vi "Main.vi"() -> ()   [LabVIEW 2017]
uses:
  1. CTL/DAQ_AO.ctl
  1. CTL/Controller.ctl
  <vilib>/Analysis/3filter.llb/Filter Passband Type.ctl
  <vilib>/DAQmx/read.llb/DAQmx Read (Analog 1D DBL 1Chan NSamp).vi
  <vilib>/DAQmx/write.llb/DAQmx Write (Digital Bool 1Line 1Point).vi
  <vilib>/DAQmx/write.llb/DAQmx Write (Analog 2D DBL NChan NSamp).vi
  <vilib>/DAQmx/create/channels.llb/DAQmx Create Channel (AO-Voltage-Basic).vi
  <vilib>/DAQmx/create/channels.llb/DAQmx Create Channel (AI-Voltage-Basic).vi
  <vilib>/DAQmx/configure/timing.llb/DAQmx Timing (Sample Clock).vi
  <vilib>/DAQmx/create/channels.llb/DAQmx Create Channel (DO-Digital Output).vi
  <vilib>/DAQmx/miscellaneous.llb/DAQmx Fill In Error Info.vi
  <vilib>/Analysis/2dsp.llb/1D Cross Correlation (DBL).vi
  <vilib>/measure/maspectr.llb/FFT Power Spectrum and PSD for 1 Chan.vi
  <vilib>/Analysis/3filter.llb/FIR Windowed Filter (DBL).vi
  <vilib>/Analysis/NI_AALPro.lvlib
  <vilib>/measure/NI_MAPro.lvlib
  <vilib>/Analysis/NI_AALBase.lvlib
panel:
  out "신호처리[1,-1][최대값":dbl
  out "신호처리[1.-1][필터후]":waveform(dbl)(graph)
  out "신호처리[1,-1,][필터후 주파수]":cluster{"f0":dbl, "df":dbl, "magnitude":dbl[]}(graph)
  out "신호처리[1,-1,][주파수]":cluster{"f0":dbl, "df":dbl, "magnitude":dbl[]}(graph)
  out "신호처리[1.-1]":waveform(dbl)(graph)
  in  "Tab Control":T1(tab)
  in  "Version Check":bool=TRUE
  in  "일시 정지 버튼":bool
  out "수신 신호 파형":waveform(dbl)(graph)
  out "송신 신호생성 파형":waveform(dbl)[](graph)
  out "신호처리파형":waveform(dbl)(graph)
  out "최대값":dbl
  out "이전 최대값":dbl
  out "최대값 차이":dbl
  in  "정지 버튼":bool
  in  "수동시작 버튼":bool
  in  "자동시작 버튼":bool
  in  "Chip_rate_Threshold":u32(knob)=10 scale=0.0..20.0
  in  "Threshold":u32(knob)=10 scale=0.0..20.0
  in  "수신시간":dbl=0.5
  in  "Rc":dbl=5500.0 min=4000.0 step=100.0
  in  "Mask 데이터 참조 경로":string="C:\\Users\\FishingNetID\\Desktop\\TRX_CONTROLLER_SIMULATRO_1.4\\3. TDMS\\Coef8.tdms"
  in  "TX_Period":dbl=3.0
  in  "Mask 길이":enum16{"8 Order", "12 Order"}(ring)
  in  "주소":string="192.168.0.147"
  in  "원격 포트 또는 서비스 이름":u16=10000
  out "원소":T2
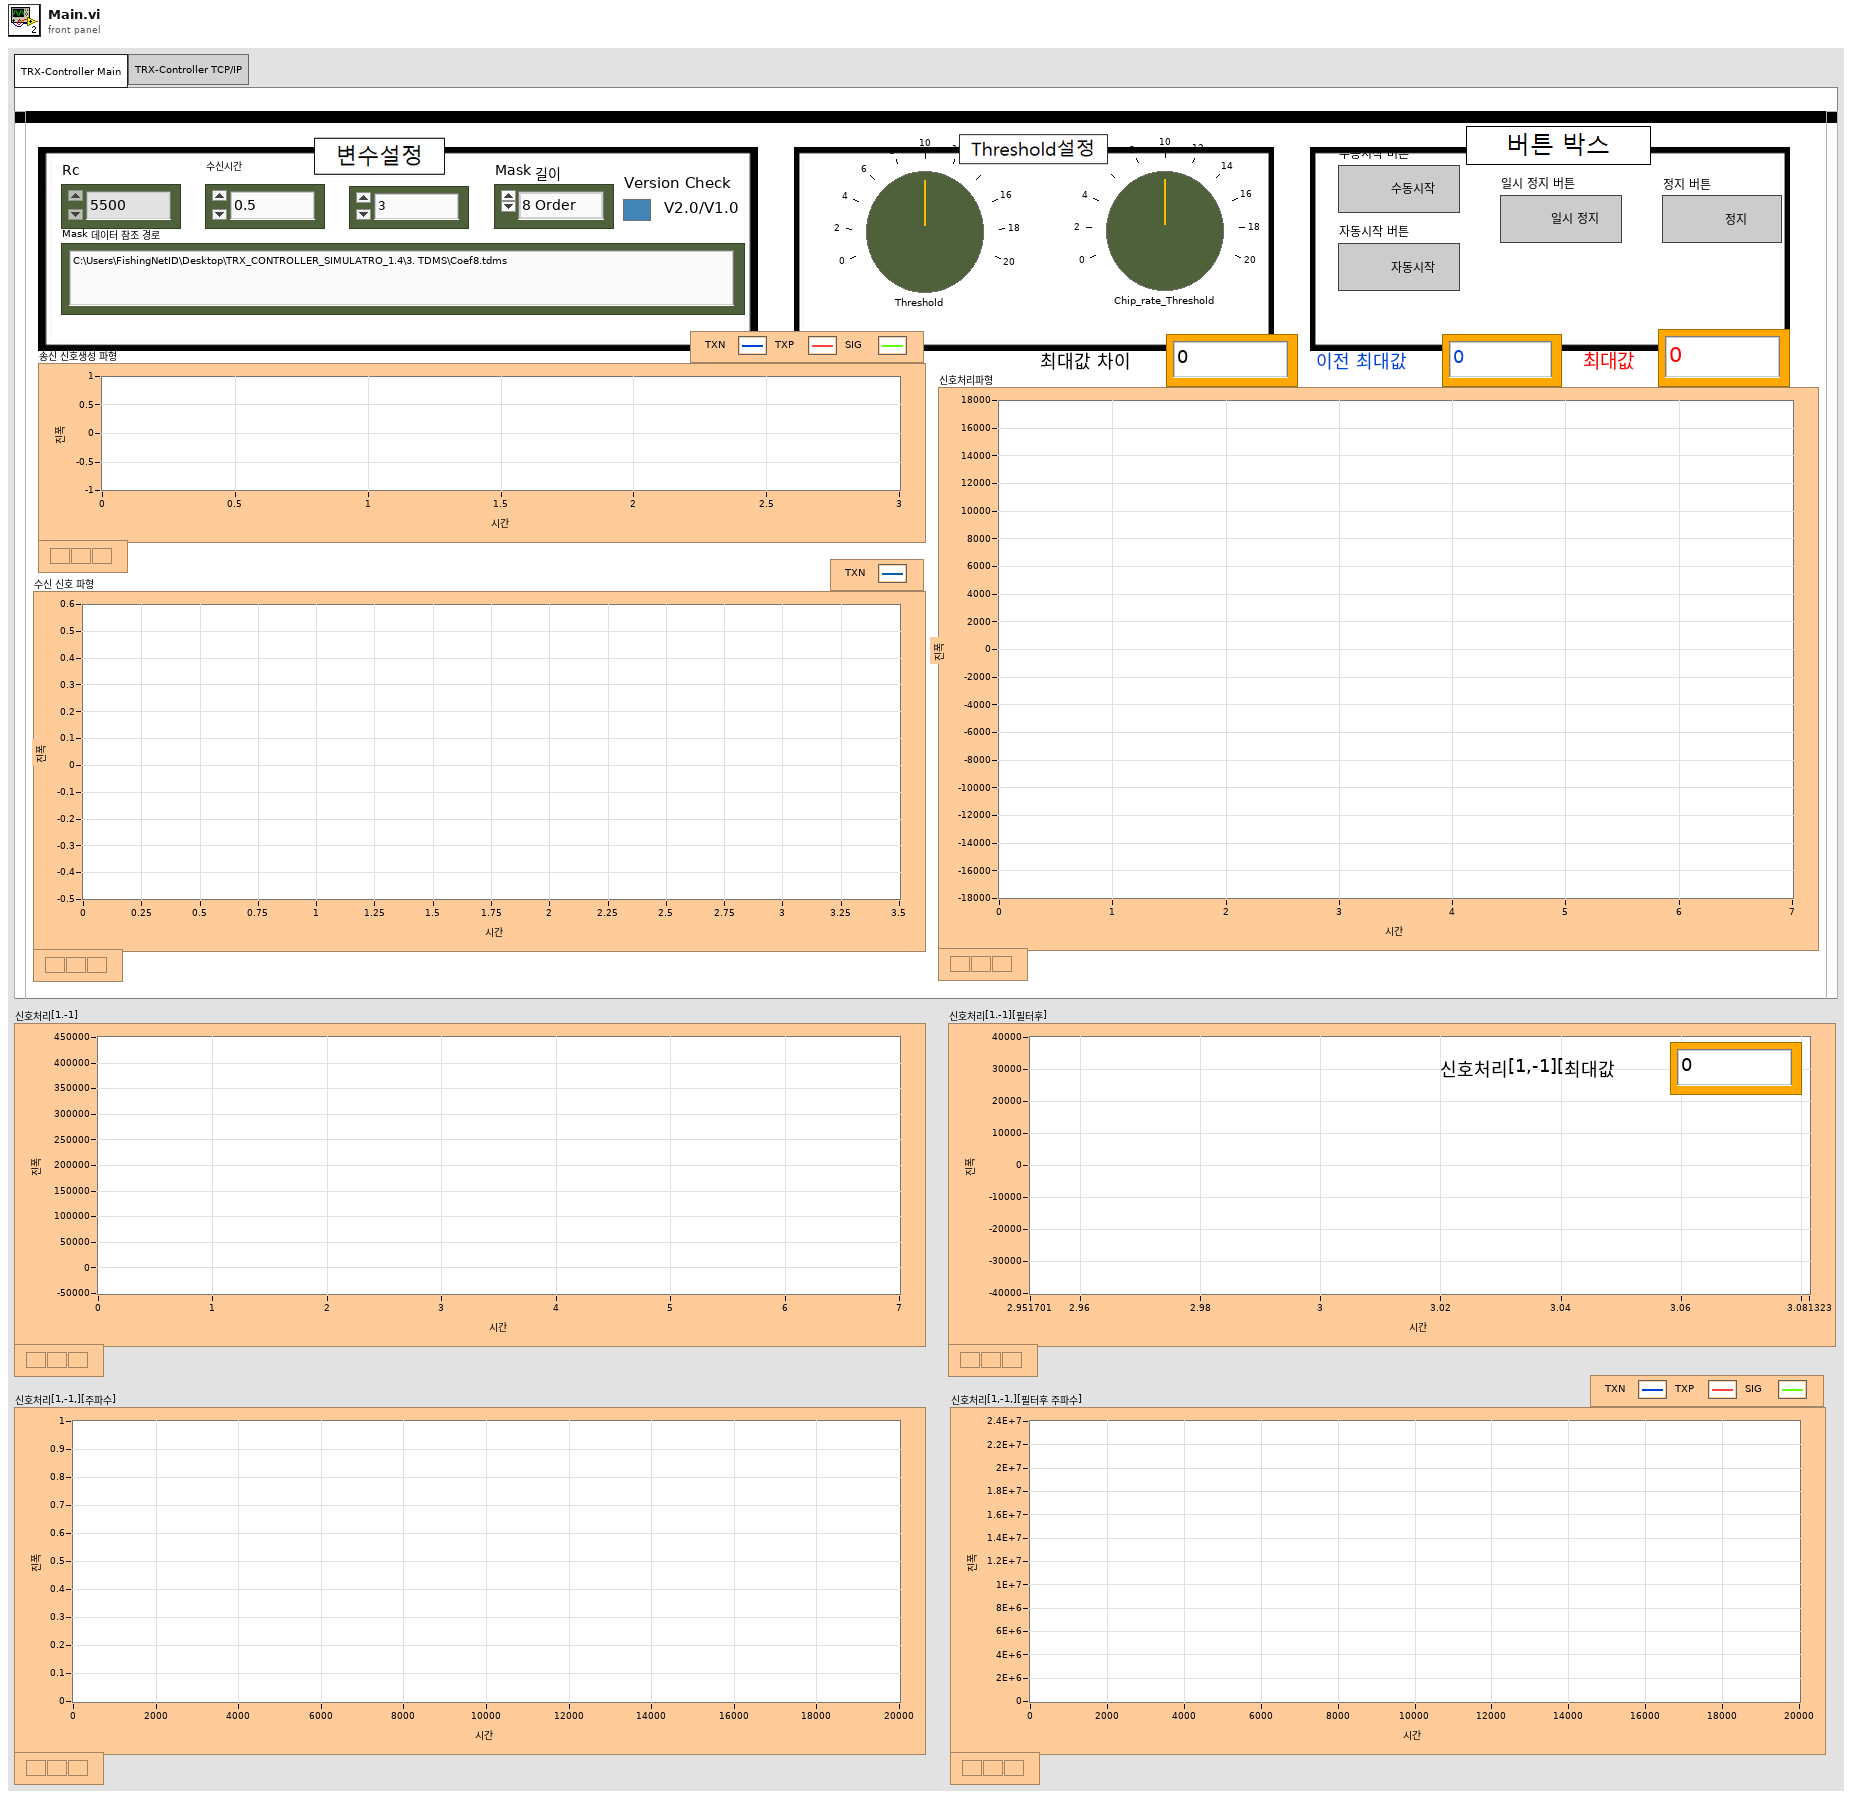
[diagram p1: front panel]
types:
  T1 = enum32{"TRX-Controller Main", "TRX-Controller TCP/IP"}
  T2 = typedef "DAQ_AO.ctl" = enum16{"통신 초기화", "통신 시작", "통신 정지"}
  T3 = cluster{"연결 ID":refnum<k5>, "TCP 에러":errorcluster}
  T4 = cluster{"송신신호 생성":waveform(dbl)[], "TXP 신호":dbl[], "TXN 신호":dbl[], "Fs":dbl, "AI 참조":refnum<k21>, "AO 참조":refnum<k21>, "수신시간":dbl, "Rc":dbl, "이전 최대값":dbl, "수신 신호처리 파형":waveform(dbl), "수신 파형":waveform(dbl), "최대값":dbl, "최대값 차이":dbl, "DO 참조":refnum<k21>, "TXEN 신호":bool[], " 신호처리[1,-1]":waveform(dbl), " 신호처리[1,-1][최대값":dbl, " 신호처리[1,-1][주파수]":cluster{"f0":dbl, "df":dbl, "magnitude":dbl[]}, " 신호처리[1,-1][필터 후 주파수]":cluster{"f0":dbl, "df":dbl, "magnitude":dbl[]}, " 신호처리[1,-1][필터후]":waveform(dbl)}
  T5 = typedef "Controller.ctl" = enum16{"초기화", "수동시작", "신호처리", "정지", "값 변경", "일시정지", "자동시작"}
  T6 = typedef "NI_AALBase.lvlib/Filter Passband Type.ctl" = enum32{"Lowpass", "Highpass", "Bandpass", "Bandstop"}
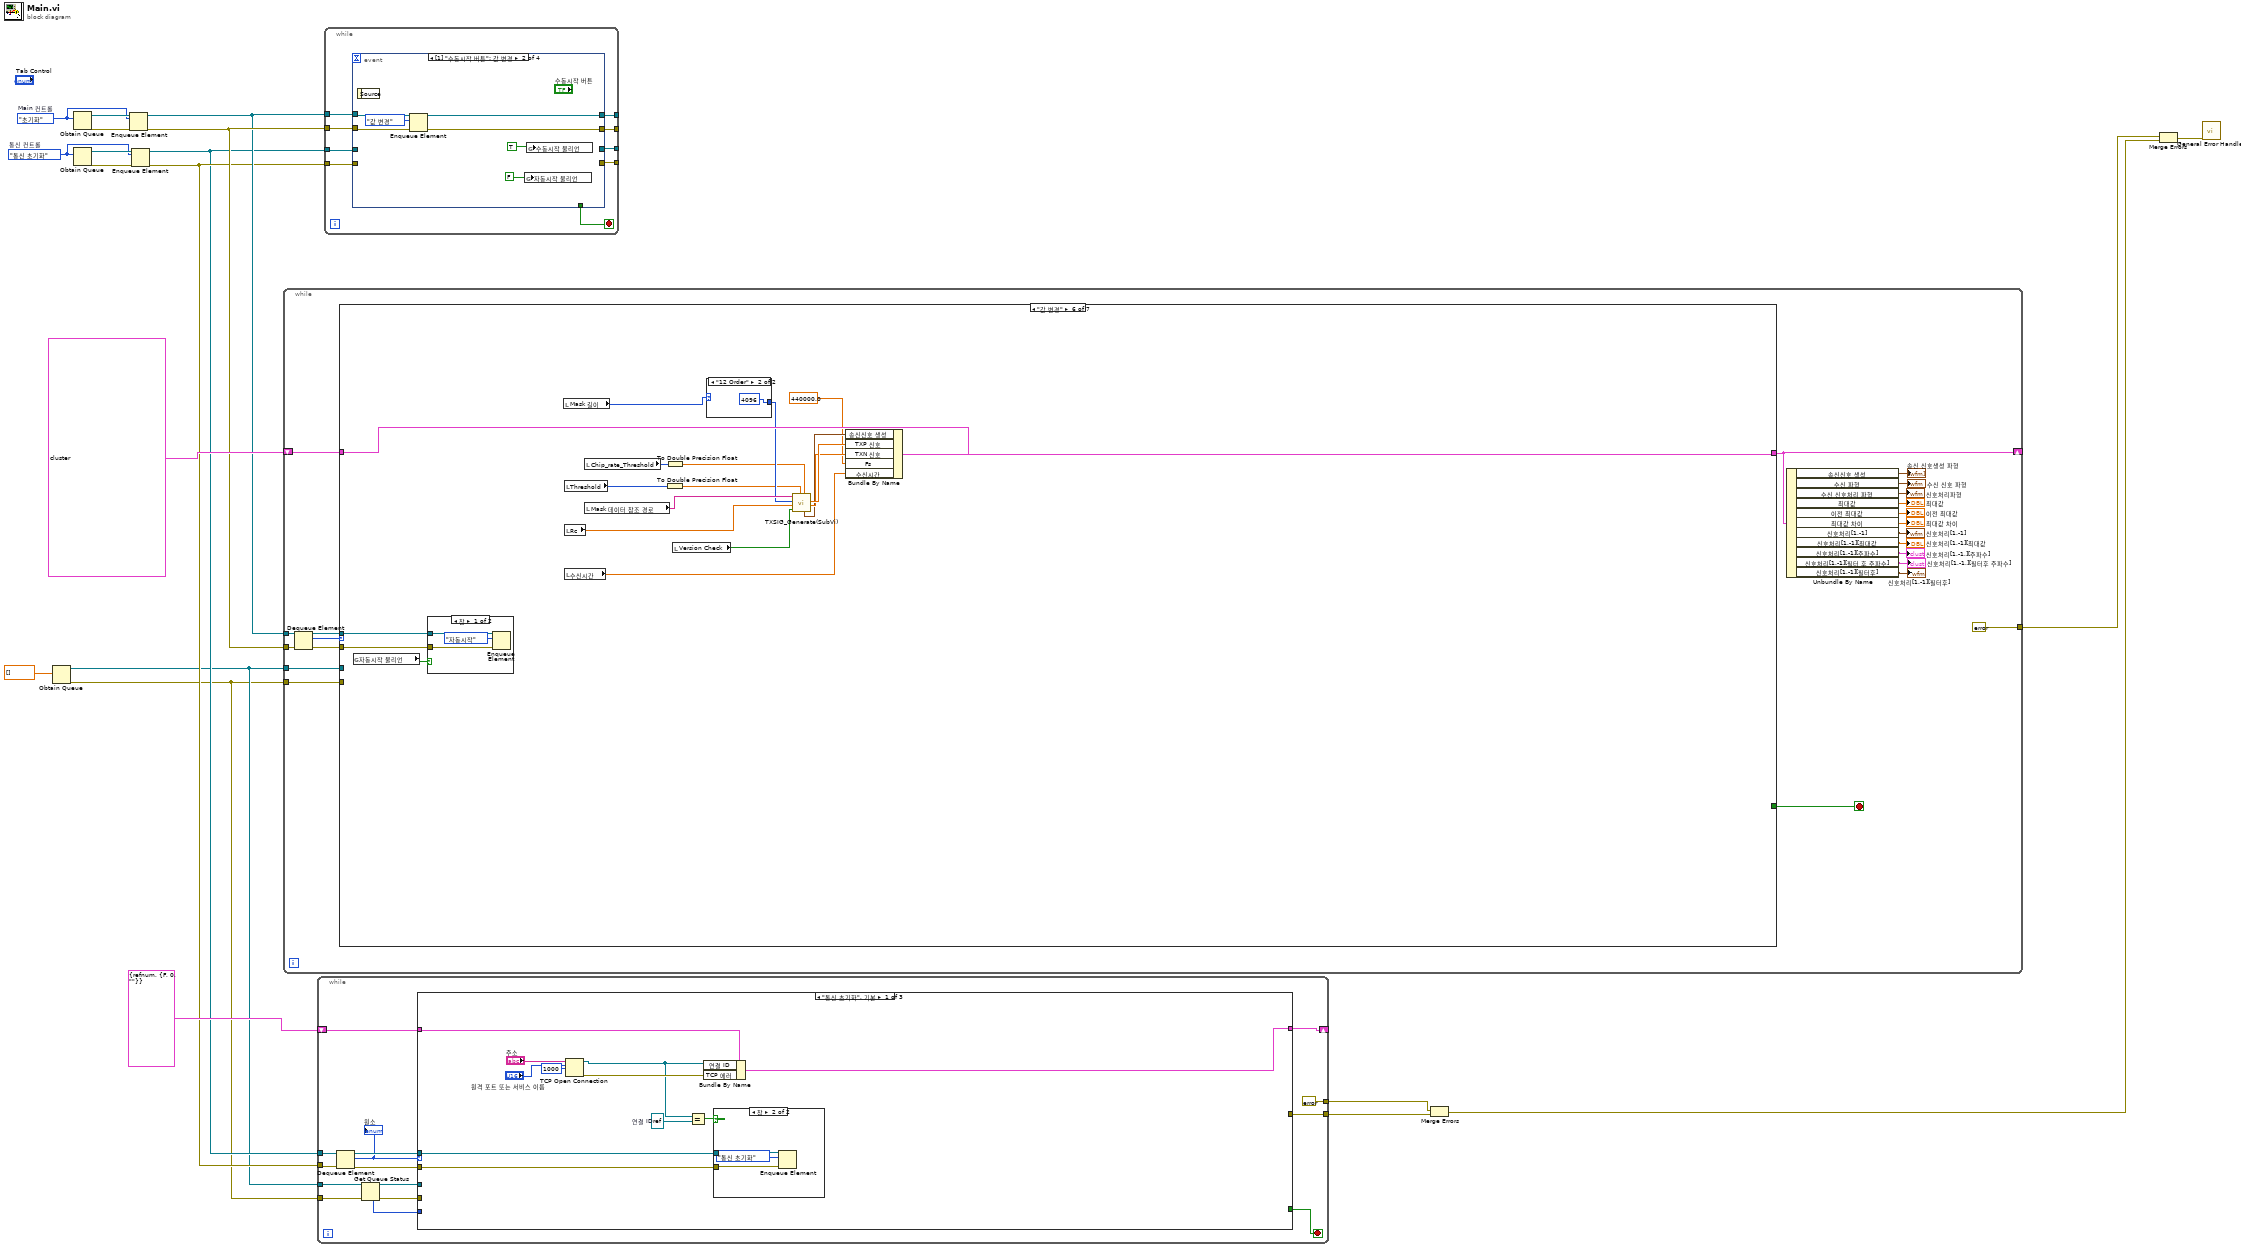
[diagram p0: block diagram]
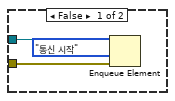
[diagram p2: hidden frame]
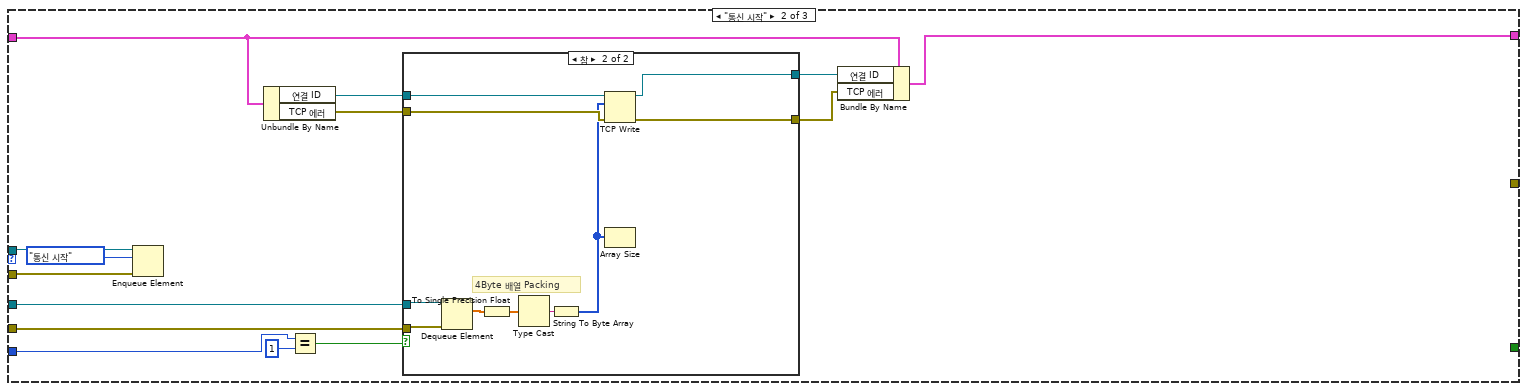
[diagram p3: hidden frame]
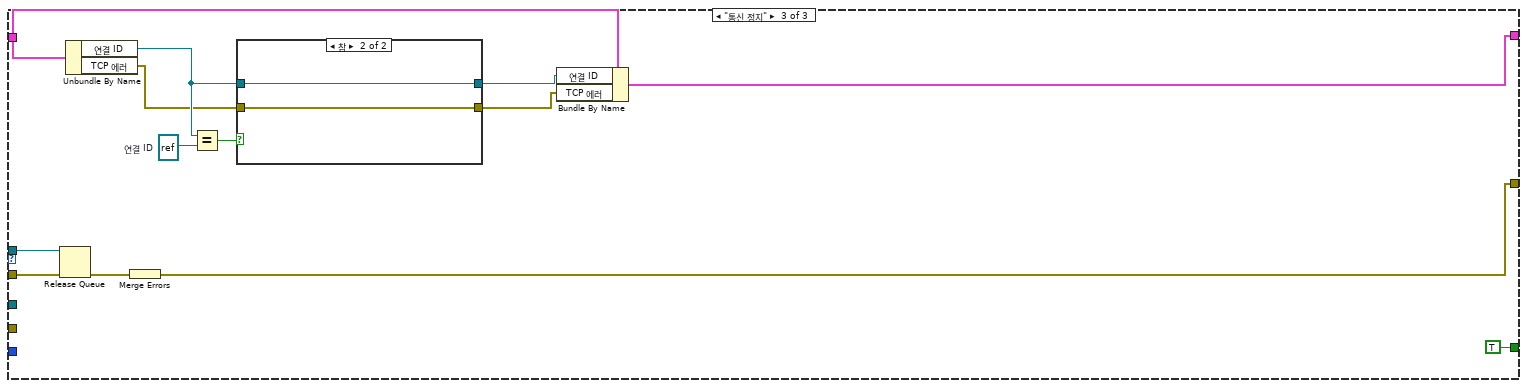
[diagram p5: hidden frame]
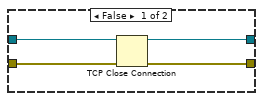
[diagram p6: hidden frame]
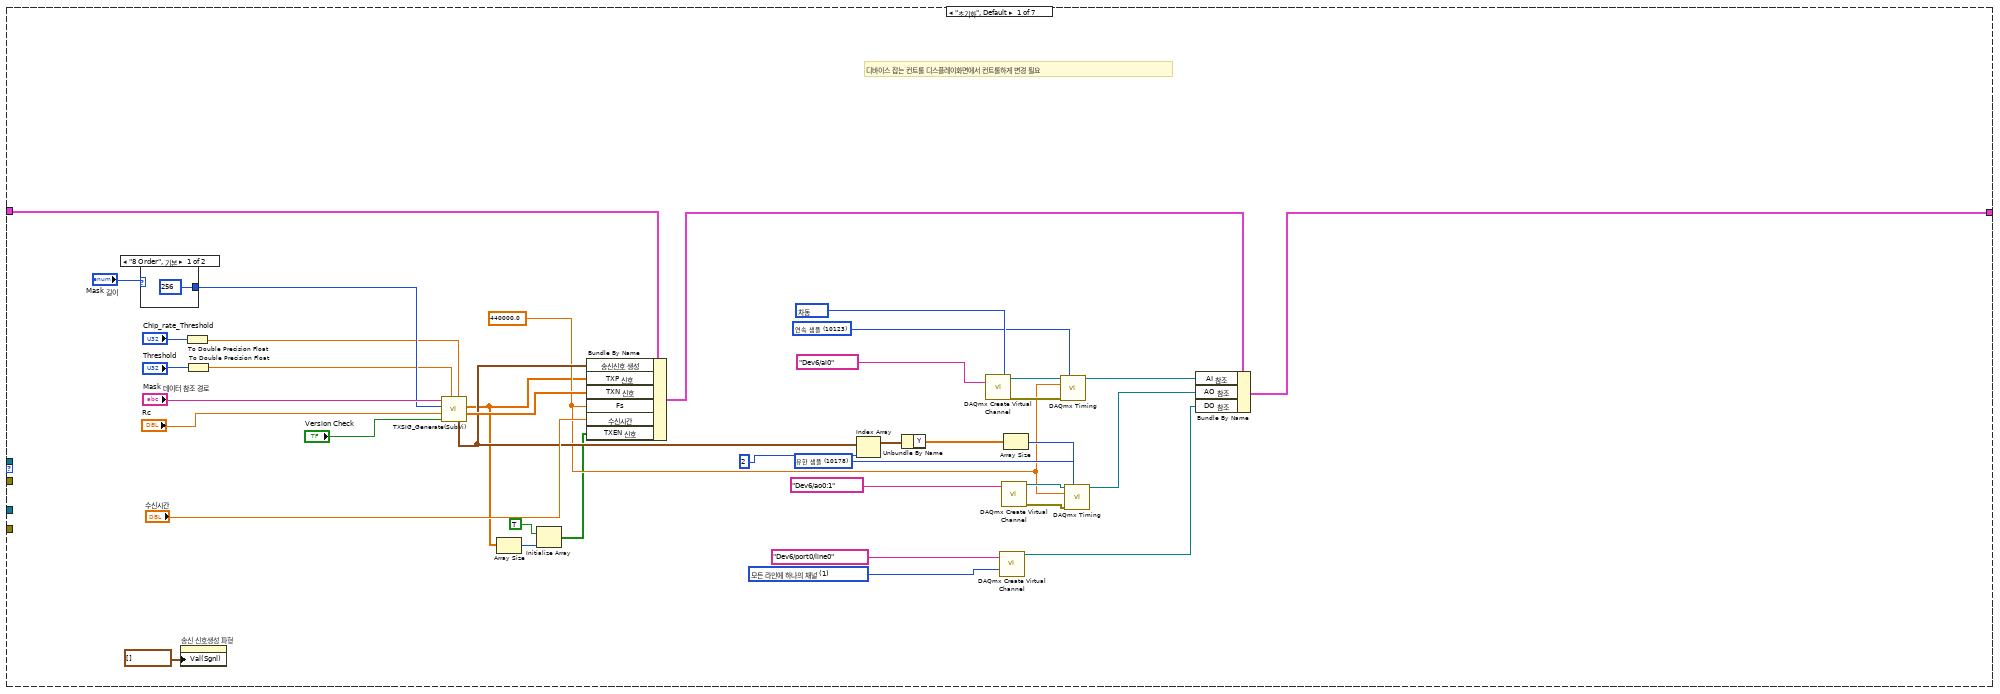
[diagram p7: hidden frame]
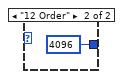
[diagram p8: hidden frame]
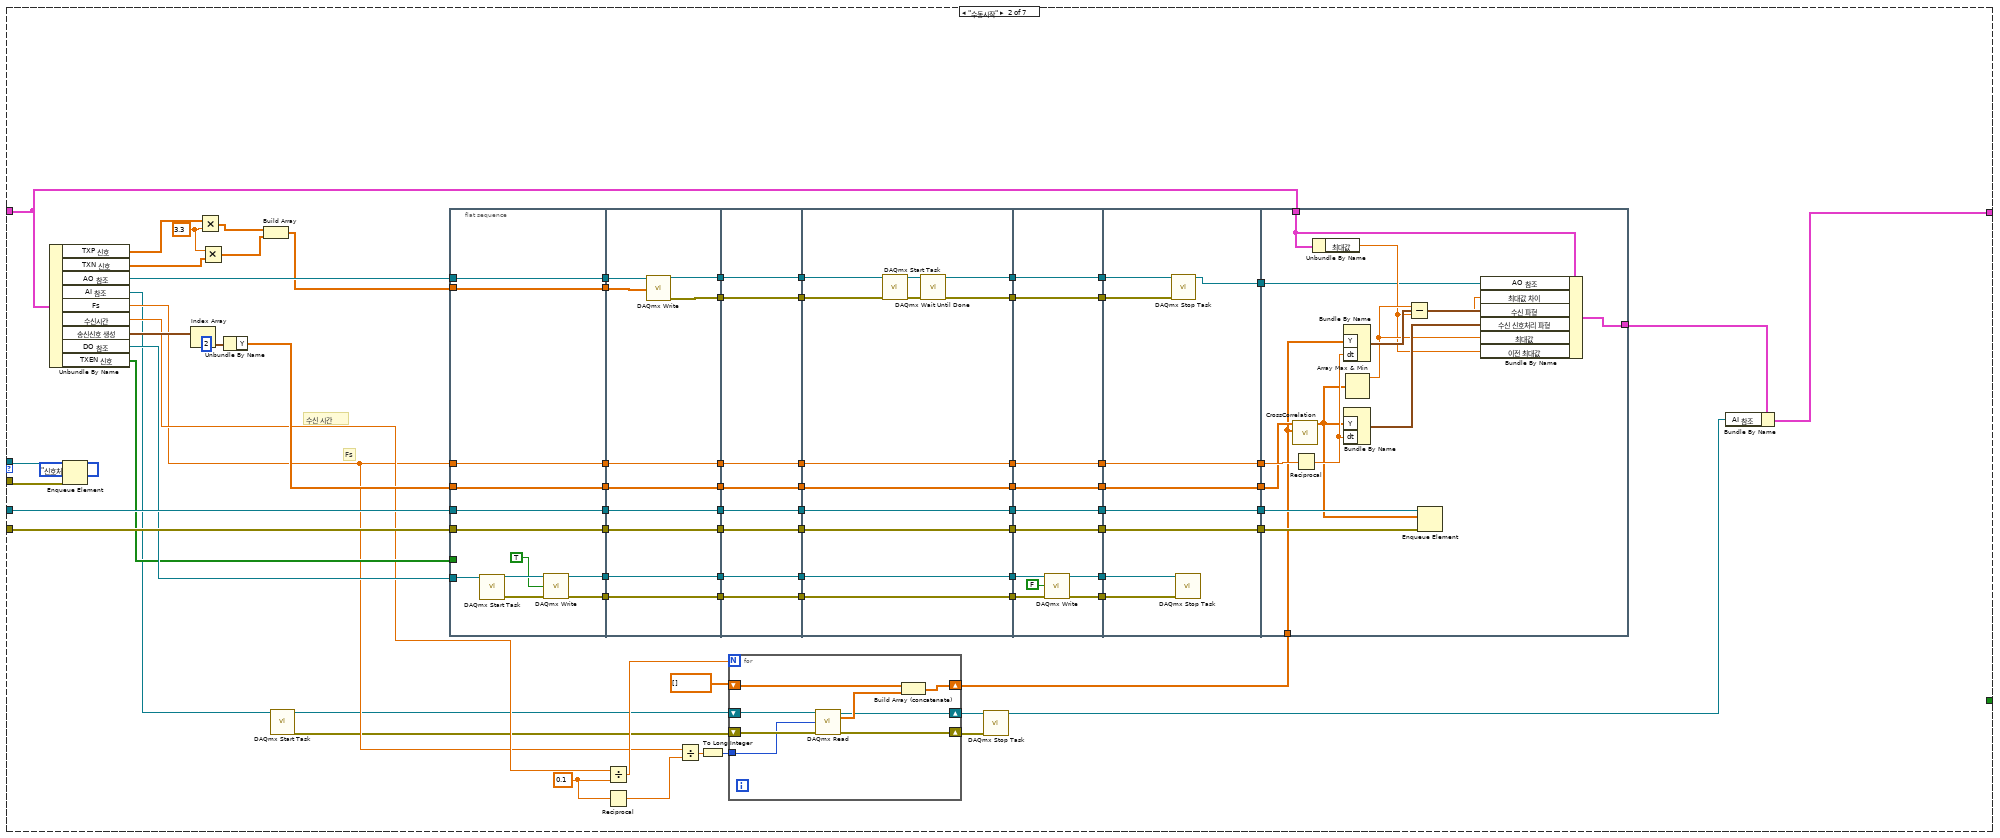
[diagram p9: hidden frame]
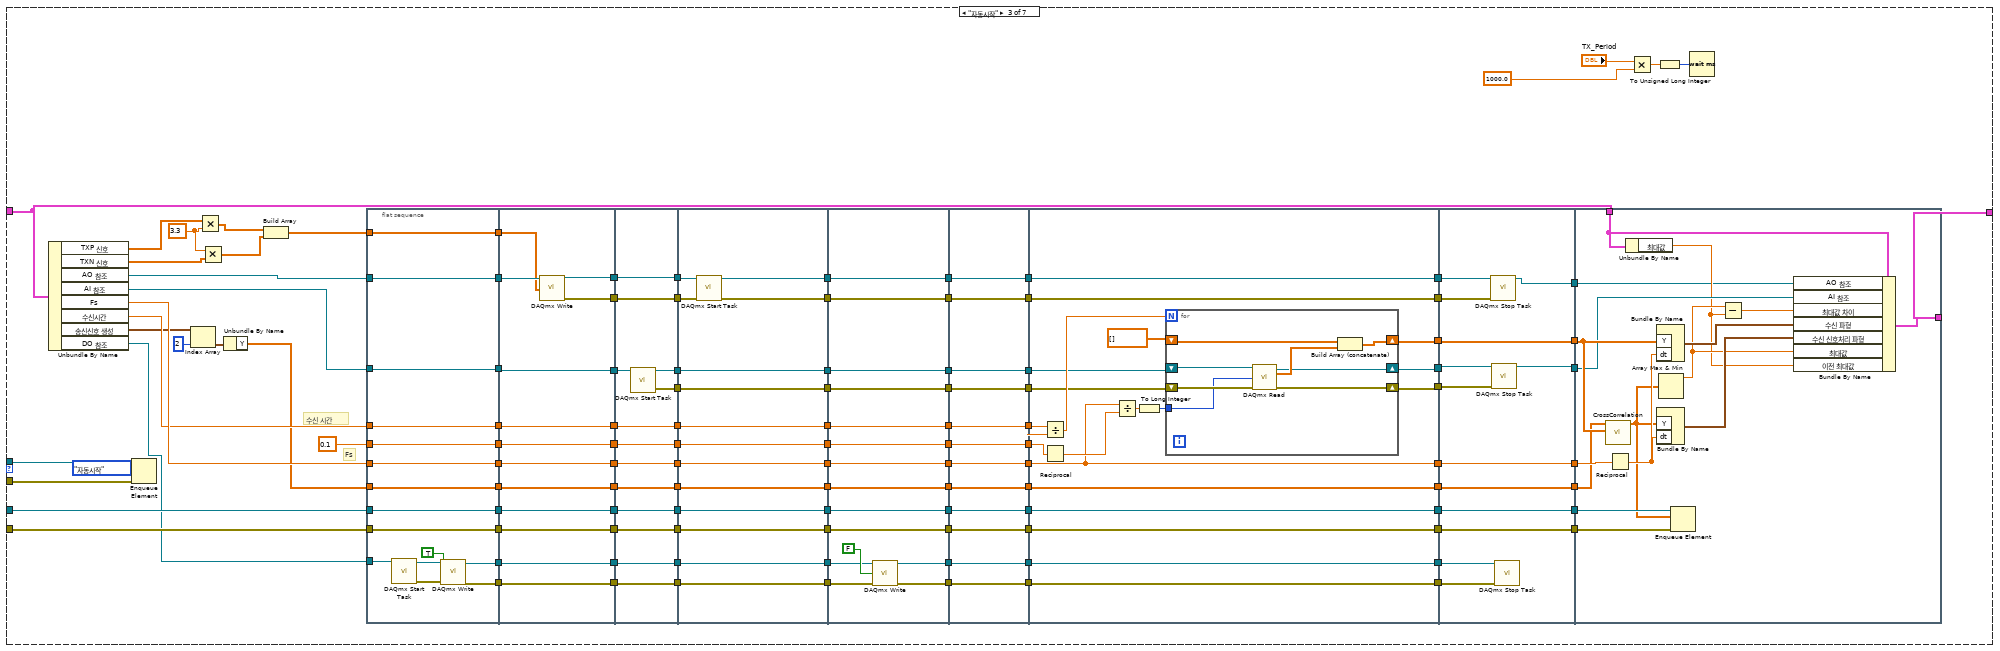
[diagram p10: hidden frame]
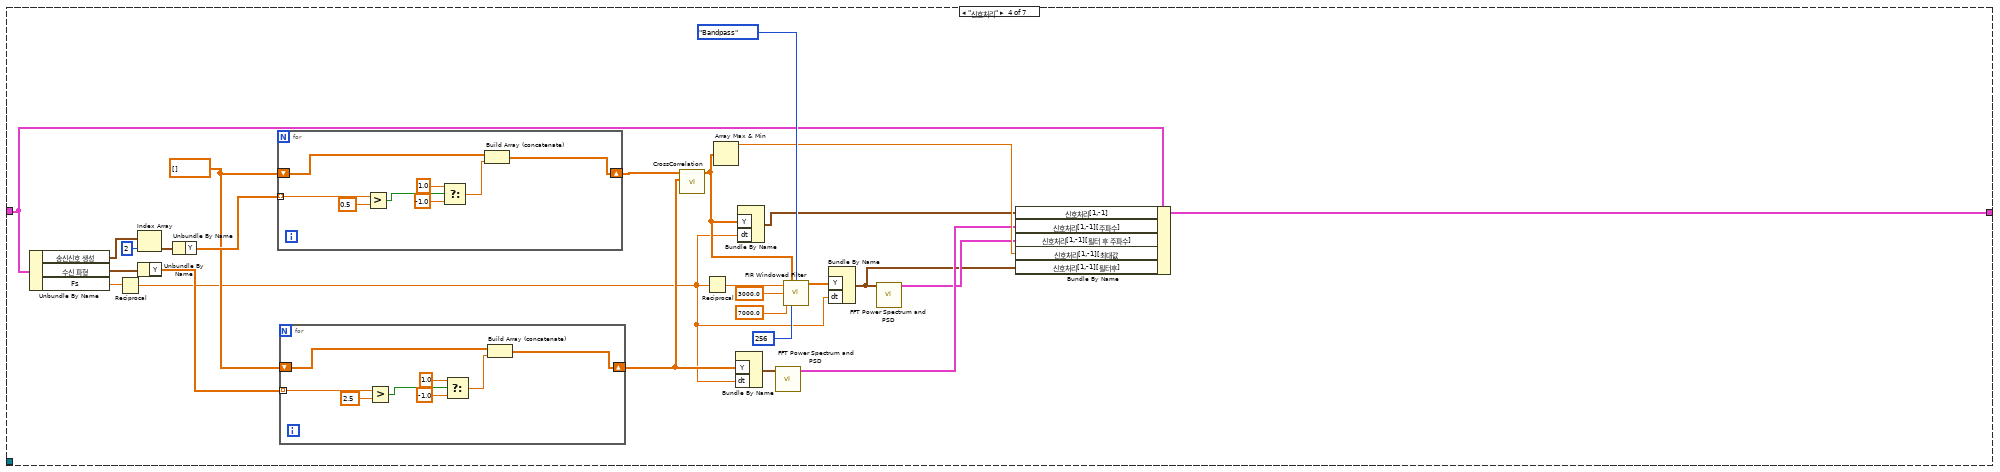
[diagram p11: hidden frame]
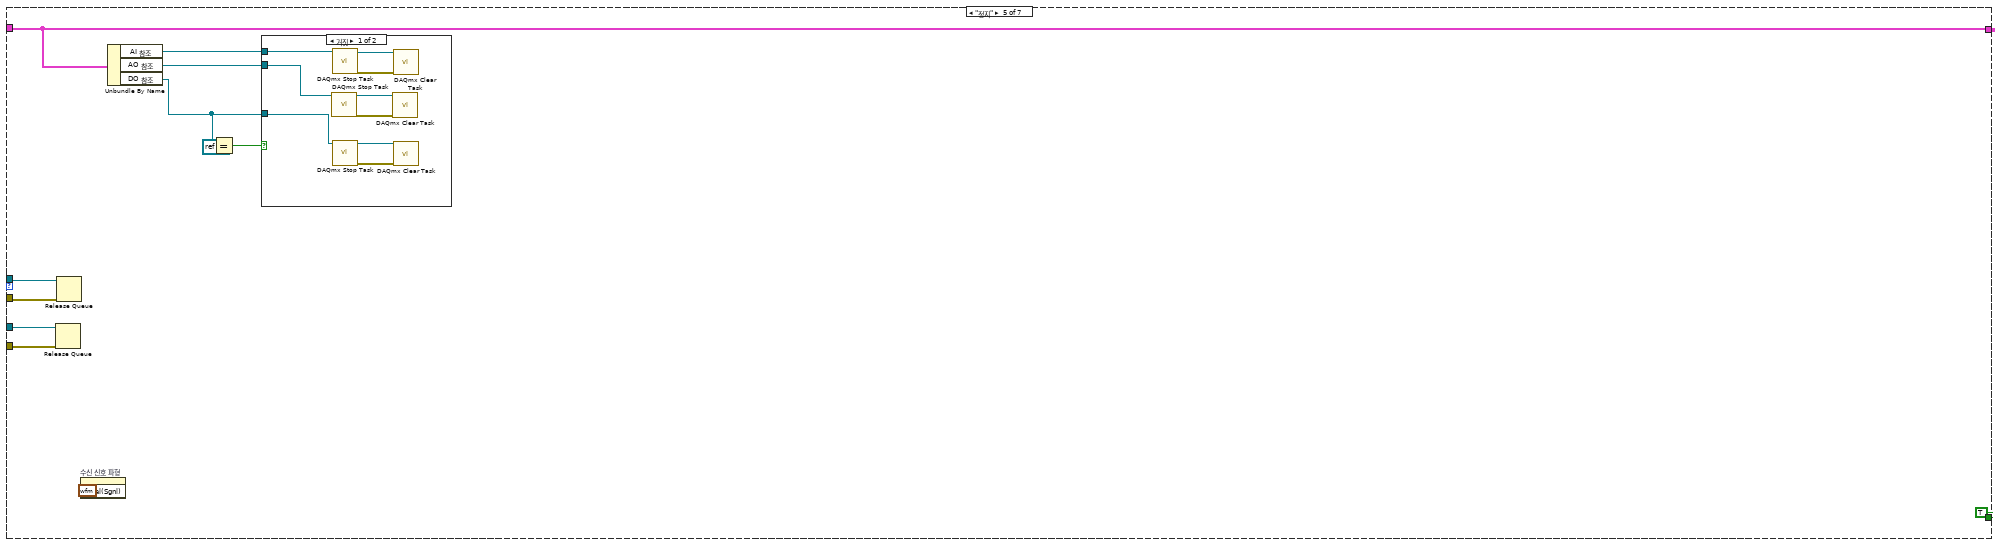
[diagram p12: hidden frame]
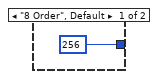
[diagram p14: hidden frame]
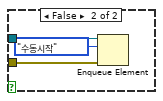
[diagram p15: hidden frame]
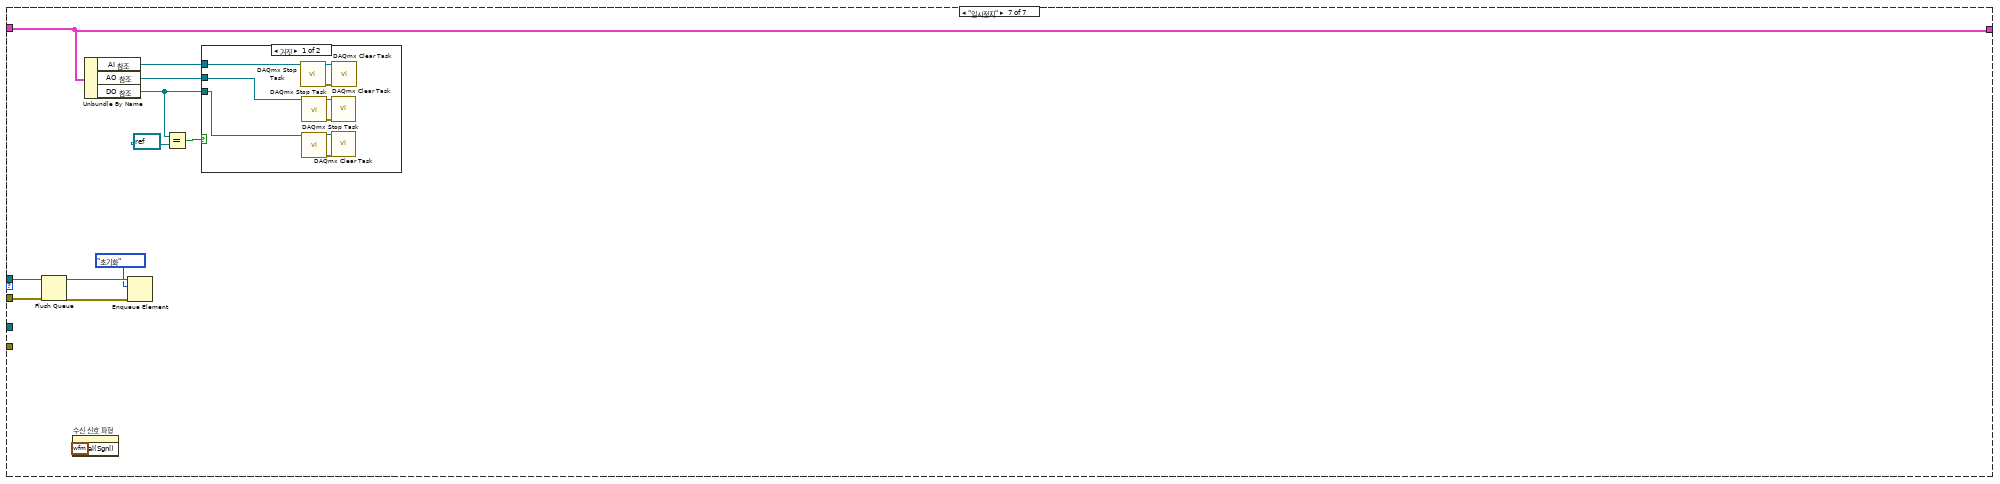
[diagram p16: hidden frame]
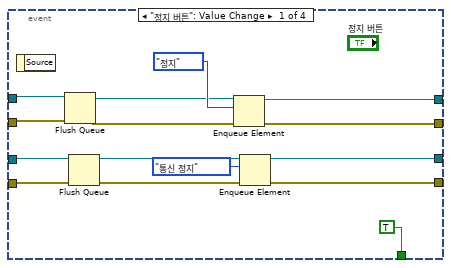
[diagram p18: hidden frame]
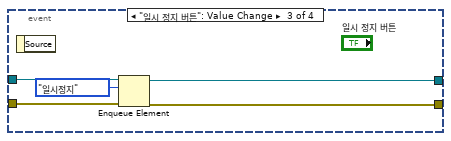
[diagram p19: hidden frame]
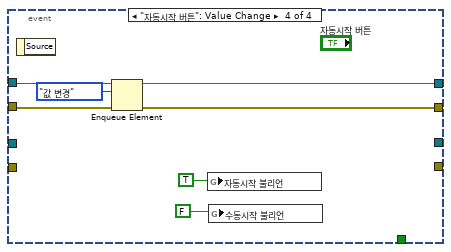
[diagram p20: hidden frame]
diagram:
  w8 = DAQ_AO."통신 초기화"  # 통신 컨트롤
  w15 = Controller."초기화"  # Main 컨트롤
  n1 = Obtain Queue(element data type=dbl[] []) -> (queue out=w2:refnum<queue>, error out=w1:errorcluster)  [unwired: 4 in, 1 out]
  n2 = Obtain Queue(element data type=w8) -> (queue out=w12:refnum<queue>, error out=w11:errorcluster)  [unwired: 4 in, 1 out]
  n3 = Obtain Queue(element data type=w15) -> (queue out=w19:refnum<queue>, error out=w18:errorcluster)  [unwired: 4 in, 1 out]
  n4 = Enqueue Element(queue=w19, element=w15, error in (no error)=w18) -> (queue out=w16:refnum<queue>, error out=w17:errorcluster)  [unwired: 1 in, 1 out]
  n5 = Enqueue Element(queue=w12, element=w8, error in (no error)=w11) -> (queue out=w9:refnum<queue>, error out=w10:errorcluster)  [unwired: 1 in, 1 out]
  n6 = while {
    tunnel: w16 -> [w42]
    tunnel: w17 -> [w41]
    tunnel: [errorcluster {"status"=FALSE, "code"=0, "source"=""} ("에러 상수")] -> w3
    shift-right: [w35] -> _
    shift-left: T4 {"송신신호 생성"=[], "TXP 신호"=[], "TXN 신호"=[], "Fs"=0.0, "AI 참조"="", "AO 참조"="", "수신시간"=0.0, "Rc"=0.0, "이전 최대값"=0.0, "수신 신호처리 파형"={"t0"=timestamp(0 s since 1904-01-01), "dt"=1.0, "Y"=[]}, "수신 파형"={"t0"=timestamp(0 s since 1904-01-01), "dt"=1.0, "Y"=[]}, "최대값"=0.0, "최대값 차이"=0.0, "DO 참조"="", "TXEN 신호"=[], " 신호처리[1,-1]"={"t0"=timestamp(0 s since 1904-01-01), "dt"=1.0, "Y"=[]}, " 신호처리[1,-1][최대값"=0.0, " 신호처리[1,-1][주파수]"={"f0"=0.0, "df"=0.0, "magnitude"=[]}, " 신호처리[1,-1][필터 후 주파수]"={"f0"=0.0, "df"=0.0, "magnitude"=[]}, " 신호처리[1,-1][필터후]"={"t0"=timestamp(0 s since 1904-01-01), "dt"=1.0, "Y"=[]}} -> [w36]
    tunnel: w2 -> [w28]
    tunnel: w1 -> [w27]
    stop <- w39 stop-if-true
    n7 = Dequeue Element(queue=w42, error in (no error)=w41) -> (queue out=w38:refnum<queue>, element=w26:T5, error out=w37:errorcluster)  [unwired: 1 in, 1 out]
    n8 = case shown="\"값 변경\"" w26 {
      tunnel: [_ _ _ _ TRUE _ _] -> w39
      tunnel: w36 -> [w78 w163 w357 w511 w556 w577 w599]
      tunnel: [w79 w86 w336 w510 w556 w581 w599] -> w35
      tunnel: w38 -> [_ w126 w335 _ w547 w579 w605]
      tunnel: w37 -> [_ w125 w334 _ w546 w578 w604]
      tunnel: w28 -> [_ w153 w332 _ w549 _ _]
      tunnel: w27 -> [_ w151 w331 _ w548 _ _]
      frame "초기화", Default {
        w49 = 1 items=["각 라인에 하나의 채널", "모든 라인에 하나의 채널"] ("line grouping")
        w51 = 440000.0 ("Fs")
        w76 = 10106 items=["기본"=-1, "RSE"=10083, "NRSE"=10078, "차동"=10106, "유사 차동"=12529] ("input terminal configuration")
        w70 = 10178 items=["유한 샘플"=10178, "연속 샘플"=10123, "하드웨어 타이밍에 의한 단일 포인트"=12522] ("sample mode")
        w73 = 10123 items=["유한 샘플"=10178, "연속 샘플"=10123, "하드웨어 타이밍에 의한 단일 포인트"=12522] ("sample mode")
        # "디바이스 잡는 컨트롤 디스플레이화면에서 컨트롤하게 변경 필요"
        n9 = case shown="\"8 Order\", 기본" "Mask 길이" {
          tunnel: [256 4096] -> w61
          frame "8 Order", Default {
          }
          frame "12 Order" {
          }
        }
        n10 = property on="송신 신호생성 파형" class="WFGraph (엄격한)"("Val(Sgnl)"=waveform(dbl)[] []) -> ()  [unwired: 2 in, 2 out]
        n11 = To Double Precision Float(number="Chip_rate_Threshold") -> (double precision float=w59:dbl)
        n12 = To Double Precision Float(number="Threshold") -> (double precision float=w57:dbl)
        n13 = call "TXSIG_Generate(SubVi).vi"("Chip_rate_Threshold"=w59, "ThresHold"=w57, "Version 스위치"="Version Check", "Rc"="Rc", "길이"=w61, "이름 또는 상대 경로"="Mask 데이터 참조 경로") -> ("TXN"=w65:dbl[], "TXP"=w47:dbl[], "TXSIG"=w53:waveform(dbl)[])  [unwired: 3 in]
        n14 = Array Size(array=w47) -> (size(s)=w46:i32)
        n15 = Initialize Array(TRUE, w46) -> (w44:bool[])
        n16 = Bundle By Name(cluster=w78, "송신신호 생성"=w53, "TXP 신호"=w47, "TXN 신호"=w65, "Fs"=w51, "수신시간"="수신시간", "TXEN 신호"=w44) -> (w77:T4)
        n17 = Index Array(array=w53, index=2 ("인덱스")) -> (element=w55:waveform(dbl))
        n18 = Unbundle By Name(w55) -> ("Y"=w54:dbl[])
        n19 = call-poly <vilib>:"DAQmx Create Virtual Channel.vi"("input terminal configuration"=w76, "physical channels"=tag "Dev6/ai0") -> ("task out"=w75:refnum<k21>, "error out"=w74:errorcluster)  [unwired: 12 in]
        n20 = call-poly <vilib>:"DAQmx Create Virtual Channel.vi"("lines"=tag "Dev6/port0/line0", "line grouping"=w49) -> ("task out"=w48:refnum<k21>)  [unwired: 12 in, 1 out]
        n21 = call-poly <vilib>:"DAQmx Create Virtual Channel.vi"("physical channels"=tag "Dev6/ao0:1") -> ("task out"=w71:refnum<k21>, "error out"=w68:errorcluster)  [unwired: 13 in]
        n22 = Array Size(array=w54) -> (size(s)=w67:i32)
        n23 = call-poly <vilib>:"DAQmx Timing.vi"("task/channels in"=w75, "sample mode"=w73, "rate"=w51, "error in"=w74) -> ("task out"=w72:refnum<k21>)  [unwired: 10 in, 1 out]
        n24 = call-poly <vilib>:"DAQmx Timing.vi"("task/channels in"=w71, "sample mode"=w70, "samples per channel"=w67, "rate"=w51, "error in"=w68) -> ("task out"=w69:refnum<k21>)  [unwired: 9 in, 1 out]
        n25 = Bundle By Name(cluster=w77, "AI 참조"=w72, "AO 참조"=w69, "DO 참조"=w48) -> (w79:T4)
      }
      frame "수동시작" {
        w99 = 0.1 ("y")
        w158 = 3.3
        # "Fs"
        # "수신 시간"
        n26 = Unbundle By Name(w163) -> ("TXP 신호"=w160:dbl[], "TXN 신호"=w159:dbl[], "AO 참조"=w164:refnum<k21>, "AI 참조"=w84:refnum<k21>, "Fs"=w98:dbl, "수신시간"=w100:dbl, "송신신호 생성"=w156:waveform(dbl)[], "DO 참조"=w149:refnum<k21>, "TXEN 신호"=w133:bool[])
        n27 = Enqueue Element(queue=w126, element=Controller."신호처리" ("원소"), error in (no error)=w125) -> ()  [unwired: 1 in, 3 out]
        n28 = Index Array(array=w156, index=2 ("인덱스")) -> (element=w162:waveform(dbl))
        n29 = Multiply(x=w160, y=w158) -> (x*y=w134:dbl[])
        n30 = Multiply(x=w158, y=w159) -> (x*y=w157:dbl[])
        n31 = Unbundle By Name(w162) -> ("Y"=w106:dbl[])
        n32 = Build Array(w134, w157) -> (w85:dbl[][])
        n33 = call <vilib>:"DAQmx Start Task.vi"("task/channels in"=w84) -> ("task out"=w97:refnum<k21>, "error out"=w96:errorcluster)  [unwired: 13 in]
        n34 = flat-sequence {
          tunnel: w149 -> [w178]
          tunnel: w151 -> [w179]
          tunnel: w153 -> [w180]
          tunnel: w106 -> [w181]
          tunnel: w85 -> [w182]
          tunnel: w98 -> [w183]
          tunnel: w164 -> [w184]
          tunnel: [w184] -> w148
          tunnel: [w183] -> w147
          tunnel: [w182] -> w146
          tunnel: [w181] -> w145
          tunnel: [w180] -> w144
          tunnel: [w179] -> w143
          tunnel: [w175] -> w138
          tunnel: [w174] -> w137
          tunnel: w133 -> [_]
          tunnel: [w193] -> w109
          tunnel: [w192] -> w111
          tunnel: [w191] -> w113
          tunnel: [w189] -> w115
          tunnel: [w188] -> w117
          tunnel: [w187] -> w119
          tunnel: w148 -> [w194]
          tunnel: w147 -> [w191]
          tunnel: w146 -> [w190]
          tunnel: w145 -> [w189]
          tunnel: w144 -> [w188]
          tunnel: w143 -> [w187]
          tunnel: [w186] -> w121
          tunnel: w138 -> [w186]
          tunnel: w137 -> [w185]
          tunnel: [w185] -> w123
          tunnel: w123 -> [w202]
          tunnel: [w202] -> w122
          tunnel: w121 -> [w201]
          tunnel: [w201] -> w120
          tunnel: w119 -> [w200]
          tunnel: [w200] -> w118
          tunnel: w117 -> [w199]
          tunnel: [w199] -> w116
          tunnel: w115 -> [w198]
          tunnel: [w198] -> w114
          tunnel: w113 -> [w197]
          tunnel: [w197] -> w112
          tunnel: w111 -> [w196]
          tunnel: [w196] -> w110
          tunnel: w109 -> [w195]
          tunnel: [w195] -> w108
          tunnel: [w214] -> w132
          tunnel: [w213] -> w131
          tunnel: [w212] -> w130
          tunnel: [w211] -> w129
          tunnel: [w210] -> w128
          tunnel: [w209] -> w127
          tunnel: w122 -> [w209]
          tunnel: w120 -> [w210]
          tunnel: w118 -> [w211]
          tunnel: w116 -> [w212]
          tunnel: w114 -> [w213]
          tunnel: w112 -> [w214]
          tunnel: w110 -> [w208]
          tunnel: w108 -> [w207]
          tunnel: [w204] -> w92
          tunnel: [w203] -> w91
          tunnel: w132 -> [w225]
          tunnel: [w225] -> w142
          tunnel: w131 -> [w224]
          tunnel: [w224] -> w141
          tunnel: w130 -> [w223]
          tunnel: [w223] -> w140
          tunnel: w129 -> [w222]
          tunnel: [w222] -> w139
          tunnel: w128 -> [w221]
          tunnel: w127 -> [w220]
          tunnel: [w219] -> w136
          tunnel: [w218] -> w135
          tunnel: [w216] -> w93
          tunnel: w92 -> [w216]
          tunnel: w91 -> [w215]
          tunnel: [w215] -> w90
          tunnel: [w234] -> w155
          tunnel: [w233] -> w154
          tunnel: [w232] -> w152
          tunnel: [w231] -> w150
          tunnel: [w228] -> w107
          tunnel: w142 -> [w234]
          tunnel: w141 -> [w233]
          tunnel: w140 -> [w232]
          tunnel: w139 -> [w231]
          tunnel: w136 -> [w230]
          tunnel: w135 -> [w229]
          tunnel: w93 -> [w227]
          tunnel: w90 -> [w226]
          tunnel: w163 -> [w246]
          tunnel: w155 -> [w248]
          tunnel: w154 -> [w247]
          tunnel: [w243] -> w88
          tunnel: w152 -> [w239]
          tunnel: w150 -> [w238]
          tunnel: w107 -> [w236]
          tunnel: w89 -> [w235]
          frame #0 {
            n35 = call <vilib>:"DAQmx Start Task.vi"("task/channels in"=w178) -> ("task out"=w177:refnum<k21>, "error out"=w176:errorcluster)  [unwired: 13 in]
            n36 = call-poly <vilib>:"DAQmx Write.vi"("task/channels in"=w177, "data"=TRUE, "error in"=w176) -> ("task out"=w175:refnum<k21>, "error out"=w174:errorcluster)  [unwired: 10 in, 1 out]
          }
          frame #1 {
            n37 = call-poly <vilib>:"DAQmx Write.vi"("task/channels in"=w194, "data"=w190) -> ("task out"=w193:refnum<k21>, "error out"=w192:errorcluster)  [unwired: 11 in, 1 out]
          }
          frame #2 {
          }
          frame #3 {
            n38 = call <vilib>:"DAQmx Start Task.vi"("task/channels in"=w207, "error in"=w208) -> ("task out"=w206:refnum<k21>, "error out"=w205:errorcluster)  [unwired: 12 in]
            n39 = call <vilib>:"DAQmx Wait Until Done.vi"("task/channels in"=w206, "error in"=w205) -> ("task out"=w204:refnum<k21>, "error out"=w203:errorcluster)  [unwired: 12 in]
          }
          frame #4 {
            n40 = call-poly <vilib>:"DAQmx Write.vi"("task/channels in"=w221, "data"=FALSE, "error in"=w220) -> ("task out"=w219:refnum<k21>, "error out"=w218:errorcluster)  [unwired: 10 in, 1 out]
          }
          frame #5 {
            n41 = call <vilib>:"DAQmx Stop Task.vi"("task/channels in"=w227, "error in"=w226) -> ("task out"=w228:refnum<k21>)  [unwired: 12 in, 1 out]
            n42 = call <vilib>:"DAQmx Stop Task.vi"("task/channels in"=w230, "error in"=w229) -> ()  [unwired: 12 in, 2 out]
          }
          frame #6 {
            n43 = call-poly <vilib>:"CrossCorrelation.vi"("Y"=w235, "X"=w247) -> ("Rxy"=w237:dbl[])  [unwired: 8 in, 1 out]
            n44 = Reciprocal(x=w248) -> (1/x=w249:dbl)
            n45 = Unbundle By Name(w246) -> ("최대값"=w240:dbl)
            n46 = Bundle By Name("Y"=w235, "dt"=w249) -> (w245:waveform(dbl))  [unwired: 1 in]
            n47 = Bundle By Name("Y"=w237, "dt"=w249) -> (w244:waveform(dbl))  [unwired: 1 in]
            n48 = Array Max & Min(array=w237) -> (max value=w241:dbl)  [unwired: 3 out]
            n49 = Subtract(x=w241, y=w240) -> (x-y=w242:dbl)
            n50 = Enqueue Element(queue=w239, element=w237, error in (no error)=w238) -> ()  [unwired: 1 in, 3 out]
            n51 = Bundle By Name(cluster=w246, "AO 참조"=w236, "최대값 차이"=w242, "수신 파형"=w245, "수신 신호처리 파형"=w244, "최대값"=w241, "이전 최대값"=w240) -> (w243:T4)
          }
        }
        n52 = Divide(x=w100, y=w99) -> (x/y=w102:dbl)
        n53 = Reciprocal(x=w99) -> (1/x=w103:dbl)
        n54 = Divide(x=w98, y=w103) -> (x/y=w105:dbl)
        n55 = To Long Integer(number=w105) -> (32bit integer=w104:i32)
        n56 = for {
          N: w102 -> [_]
          shift-right: [w170] -> w89
          shift-left: dbl[] [] -> [w172]
          shift-right: [w166] -> w95
          shift-left: w97 -> [w169]
          shift-right: [w167] -> w94
          shift-left: w96 -> [w168]
          tunnel: w104 -> [w165]
          n57 = call-poly <vilib>:"DAQmx Read.vi"("task/channels in"=w169, "number of samples per channel"=w165, "error in"=w168) -> ("task out"=w166:refnum<k21>, "data"=w171:dbl[], "error out"=w167:errorcluster)  [unwired: 10 in]
          n58 = Build Array (concatenate)(w172, w171) -> (w170:dbl[])
        }
        n59 = call <vilib>:"DAQmx Stop Task.vi"("task/channels in"=w95, "error in"=w94) -> ("task out"=w87:refnum<k21>)  [unwired: 12 in, 1 out]
        n60 = Bundle By Name(cluster=w88, "AI 참조"=w87) -> (w86:T4)
      }
      frame "자동시작" {
        w349 = 3.3
        # "Fs"
        # "수신 시간"
        n61 = Unbundle By Name(w357) -> ("TXP 신호"=w351:dbl[], "TXN 신호"=w350:dbl[], "AO 참조"=w364:refnum<k21>, "AI 참조"=w345:refnum<k21>, "Fs"=w363:dbl, "수신시간"=w360:dbl, "송신신호 생성"=w346:waveform(dbl)[], "DO 참조"=w310:refnum<k21>)
        n62 = Enqueue Element(queue=w335, element=Controller."자동시작" ("원소"), error in (no error)=w334) -> ()  [unwired: 1 in, 3 out]
        n63 = Index Array(array=w346, index=2 ("인덱스")) -> (element=w353:waveform(dbl))
        n64 = Multiply(x=w351, y=w349) -> (x*y=w348:dbl[])
        n65 = Multiply(x=w349, y=w350) -> (x*y=w347:dbl[])
        n66 = Unbundle By Name(w353) -> ("Y"=w340:dbl[])
        n67 = Build Array(w348, w347) -> (w324:dbl[][])
        n68 = flat-sequence {
          tunnel: w324 -> [w371]
          tunnel: w331 -> [w372]
          tunnel: w332 -> [w373]
          tunnel: w340 -> [w374]
          tunnel: 0.1 ("y") -> [w375]
          tunnel: w360 -> [w376]
          tunnel: w363 -> [w377]
          tunnel: w345 -> [w378]
          tunnel: w364 -> [w379]
          tunnel: [w379] -> w319
          tunnel: [w378] -> w318
          tunnel: [w377] -> w317
          tunnel: [w376] -> w316
          tunnel: [w375] -> w315
          tunnel: [w374] -> w314
          tunnel: [w373] -> w313
          tunnel: [w372] -> w312
          tunnel: [w371] -> w311
          tunnel: w310 -> [w370]
          tunnel: [w366] -> w309
          tunnel: [w365] -> w307
          tunnel: [w391] -> w287
          tunnel: [w390] -> w285
          tunnel: [w389] -> w283
          tunnel: [w388] -> w281
          tunnel: [w387] -> w279
          tunnel: [w386] -> w277
          tunnel: [w385] -> w275
          tunnel: [w384] -> w273
          tunnel: w319 -> [w392]
          tunnel: w318 -> [w380]
          tunnel: w317 -> [w389]
          tunnel: w316 -> [w388]
          tunnel: w315 -> [w387]
          tunnel: w314 -> [w386]
          tunnel: w313 -> [w385]
          tunnel: w312 -> [w384]
          tunnel: w311 -> [w383]
          tunnel: w309 -> [w382]
          tunnel: [w382] -> w271
          tunnel: w307 -> [w381]
          tunnel: [w381] -> w269
          tunnel: [w380] -> w267
          tunnel: w287 -> [w405]
          tunnel: [w405] -> w286
          tunnel: w285 -> [w404]
          tunnel: [w404] -> w284
          tunnel: w283 -> [w403]
          tunnel: [w403] -> w282
          tunnel: w281 -> [w402]
          tunnel: [w402] -> w280
          tunnel: w279 -> [w401]
          tunnel: [w401] -> w278
          tunnel: w277 -> [w400]
          tunnel: [w400] -> w276
          tunnel: w275 -> [w399]
          tunnel: [w399] -> w274
          tunnel: w273 -> [w398]
          tunnel: [w398] -> w272
          tunnel: w271 -> [w397]
          tunnel: [w397] -> w270
          tunnel: w269 -> [w396]
          tunnel: [w396] -> w268
          tunnel: w267 -> [w395]
          tunnel: [w394] -> w263
          tunnel: [w393] -> w262
          tunnel: w286 -> [w413]
          tunnel: w284 -> [w412]
          tunnel: w282 -> [w419]
          tunnel: [w419] -> w361
          tunnel: [w418] -> w356
          tunnel: w280 -> [w418]
          tunnel: w278 -> [w417]
          tunnel: [w417] -> w343
          tunnel: [w416] -> w337
          tunnel: w276 -> [w416]
          tunnel: [w415] -> w328
          tunnel: w274 -> [w415]
          tunnel: [w414] -> w325
          tunnel: w272 -> [w414]
          tunnel: w270 -> [w411]
          tunnel: [w411] -> w308
          tunnel: w268 -> [w410]
          tunnel: [w410] -> w306
          tunnel: [w409] -> w264
          tunnel: w263 -> [w409]
          tunnel: w262 -> [w408]
          tunnel: [w408] -> w261
          tunnel: [w407] -> w258
          tunnel: [w406] -> w254
          tunnel: w361 -> [w434]
          tunnel: [w434] -> w303
          tunnel: [w433] -> w301
          tunnel: w356 -> [w433]
          tunnel: [w432] -> w299
          tunnel: w343 -> [w432]
          tunnel: [w431] -> w297
          tunnel: w337 -> [w431]
          tunnel: [w430] -> w295
          tunnel: w328 -> [w430]
          tunnel: [w429] -> w293
          tunnel: w325 -> [w429]
          tunnel: w308 -> [w427]
          tunnel: w306 -> [w426]
          tunnel: [w425] -> w291
          tunnel: [w424] -> w289
          tunnel: [w423] -> w265
          tunnel: w264 -> [w423]
          tunnel: w261 -> [w422]
          tunnel: [w422] -> w260
          tunnel: w258 -> [w421]
          tunnel: [w421] -> w257
          tunnel: w254 -> [w420]
          tunnel: [w420] -> w253
          tunnel: w303 -> [w446]
          tunnel: [w446] -> w302
          tunnel: w301 -> [w445]
          tunnel: [w445] -> w300
          tunnel: w299 -> [w444]
          tunnel: [w444] -> w298
          tunnel: w297 -> [w443]
          tunnel: [w443] -> w296
          tunnel: w295 -> [w442]
          tunnel: [w442] -> w294
          tunnel: w293 -> [w441]
          tunnel: [w441] -> w292
          tunnel: w291 -> [w440]
          tunnel: [w440] -> w290
          tunnel: w289 -> [w439]
          tunnel: [w439] -> w288
          tunnel: [w438] -> w266
          tunnel: w265 -> [w438]
          tunnel: w260 -> [w437]
          tunnel: [w437] -> w259
          tunnel: w257 -> [w436]
          tunnel: [w436] -> w256
          tunnel: w253 -> [w435]
          tunnel: [w435] -> w252
          tunnel: [w463] -> w362
          tunnel: w302 -> [w456]
          tunnel: w300 -> [w465]
          tunnel: [w462] -> w355
          tunnel: [w461] -> w354
          tunnel: w298 -> [w460]
          tunnel: [w456] -> w342
          tunnel: [w455] -> w338
          tunnel: w296 -> [w455]
          tunnel: [w454] -> w329
          tunnel: w294 -> [w454]
          tunnel: [w453] -> w326
          tunnel: w292 -> [w453]
          tunnel: w290 -> [w452]
          tunnel: [w452] -> w305
          tunnel: w288 -> [w451]
          tunnel: [w451] -> w304
          tunnel: w266 -> [w450]
          tunnel: w259 -> [w449]
          tunnel: w256 -> [w448]
          tunnel: [w448] -> w255
          tunnel: w252 -> [w447]
          tunnel: [w447] -> w251
          tunnel: w362 -> [w486]
          tunnel: [w485] -> w359
          tunnel: [w487] -> w358
          tunnel: w355 -> [w484]
          tunnel: w354 -> [w487]
          tunnel: w342 -> [w483]
          tunnel: [w483] -> w341
          tunnel: [w482] -> w339
          tunnel: w338 -> [w482]
          tunnel: [w481] -> w330
          tunnel: w329 -> [w481]
          tunnel: [w480] -> w327
          tunnel: w326 -> [w480]
          tunnel: w305 -> [w479]
          tunnel: w304 -> [w478]
          tunnel: w255 -> [w477]
          tunnel: w251 -> [w476]
          tunnel: [w475] -> w250
          tunnel: w357 -> [w499]
          tunnel: w341 -> [w501]
          tunnel: w358 -> [w502]
          tunnel: w359 -> [w498]
          tunnel: w339 -> [w500]
          tunnel: [w495] -> w336
          tunnel: w330 -> [w491]
          tunnel: w327 -> [w490]
          tunnel: w250 -> [w488]
          frame #0 {
            n69 = call <vilib>:"DAQmx Start Task.vi"("task/channels in"=w370) -> ("task out"=w368:refnum<k21>, "error out"=w369:errorcluster)  [unwired: 13 in]
            n70 = call-poly <vilib>:"DAQmx Write.vi"("task/channels in"=w368, "data"=TRUE, "error in"=w369) -> ("task out"=w366:refnum<k21>, "error out"=w365:errorcluster)  [unwired: 10 in, 1 out]
          }
          frame #1 {
            n71 = call-poly <vilib>:"DAQmx Write.vi"("task/channels in"=w392, "data"=w383) -> ("task out"=w391:refnum<k21>, "error out"=w390:errorcluster)  [unwired: 11 in, 1 out]
          }
          frame #2 {
            n72 = call <vilib>:"DAQmx Start Task.vi"("task/channels in"=w395) -> ("task out"=w394:refnum<k21>, "error out"=w393:errorcluster)  [unwired: 13 in]
          }
          frame #3 {
            n73 = call <vilib>:"DAQmx Start Task.vi"("task/channels in"=w413, "error in"=w412) -> ("task out"=w407:refnum<k21>, "error out"=w406:errorcluster)  [unwired: 12 in]
          }
          frame #4 {
            n74 = call-poly <vilib>:"DAQmx Write.vi"("task/channels in"=w427, "data"=FALSE, "error in"=w426) -> ("task out"=w425:refnum<k21>, "error out"=w424:errorcluster)  [unwired: 10 in, 1 out]
          }
          frame #5 {
          }
          frame #6 {
            n75 = Divide(x=w465, y=w460) -> (x/y=w464:dbl)
            n76 = Reciprocal(x=w460) -> (1/x=w459:dbl)
            n77 = Divide(x=w456, y=w459) -> (x/y=w457:dbl)
            n78 = To Long Integer(number=w457) -> (32bit integer=w458:i32)
            n79 = for {
              N: w464 -> [_]
              shift-right: [w472] -> w461
              shift-left: dbl[] [] -> [w474]
              shift-right: [w468] -> w463
              shift-left: w450 -> [w471]
              shift-right: [w469] -> w462
              shift-left: w449 -> [w470]
              tunnel: w458 -> [w467]
              n80 = call-poly <vilib>:"DAQmx Read.vi"("task/channels in"=w471, "number of samples per channel"=w467, "error in"=w470) -> ("task out"=w468:refnum<k21>, "data"=w473:dbl[], "error out"=w469:errorcluster)  [unwired: 10 in]
              n81 = Build Array (concatenate)(w474, w473) -> (w472:dbl[])
            }
          }
          frame #7 {
            n82 = call <vilib>:"DAQmx Stop Task.vi"("task/channels in"=w477, "error in"=w476) -> ("task out"=w475:refnum<k21>)  [unwired: 12 in, 1 out]
            n83 = call <vilib>:"DAQmx Stop Task.vi"("task/channels in"=w486, "error in"=w484) -> ("task out"=w485:refnum<k21>)  [unwired: 12 in, 1 out]
            n84 = call <vilib>:"DAQmx Stop Task.vi"("task/channels in"=w479, "error in"=w478) -> ()  [unwired: 12 in, 2 out]
          }
          frame #8 {
            n85 = call-poly <vilib>:"CrossCorrelation.vi"("Y"=w502, "X"=w500) -> ("Rxy"=w489:dbl[])  [unwired: 8 in, 1 out]
            n86 = Reciprocal(x=w501) -> (1/x=w503:dbl)
            n87 = Unbundle By Name(w499) -> ("최대값"=w492:dbl)
            n88 = Bundle By Name("Y"=w502, "dt"=w503) -> (w497:waveform(dbl))  [unwired: 1 in]
            n89 = Bundle By Name("Y"=w489, "dt"=w503) -> (w496:waveform(dbl))  [unwired: 1 in]
            n90 = Array Max & Min(array=w489) -> (max value=w493:dbl)  [unwired: 3 out]
            n91 = Enqueue Element(queue=w491, element=w489, error in (no error)=w490) -> ()  [unwired: 1 in, 3 out]
            n92 = Subtract(x=w493, y=w492) -> (x-y=w494:dbl)
            n93 = Bundle By Name(cluster=w499, "AO 참조"=w488, "AI 참조"=w498, "최대값 차이"=w494, "수신 파형"=w497, "수신 신호처리 파형"=w496, "최대값"=w493, "이전 최대값"=w492) -> (w495:T4)
          }
        }
        n94 = Multiply(x="TX_Period", y=1000.0) -> (x*y=w322:dbl)
        n95 = To Unsigned Long Integer(number=w322) -> (unsigned 32bit integer=w320:u32)
        n96 = Wait (ms)(milliseconds to wait=w320) -> ()  [unwired: 1 out]
      }
      frame "신호처리" {
        w524 = dbl[] []
        n97 = Unbundle By Name(w511) -> ("송신신호 생성"=w529:waveform(dbl)[], "수신 파형"=w526:waveform(dbl), "Fs"=w519:dbl)
        n98 = Reciprocal(x=w519) -> (1/x=w504:dbl)
        n99 = Index Array(array=w529, index=2 ("인덱스")) -> (element=w527:waveform(dbl))
        n100 = Unbundle By Name(w526) -> ("Y"=w523:dbl[])
        n101 = Unbundle By Name(w527) -> ("Y"=w525:dbl[])
        n102 = for {
          shift-right: [w538] -> w522
          shift-left: w524 -> [w545]
          tunnel: w525 -> [w544] mode=indexing
          n103 = Greater?(x=w544, y=0.5) -> (0:w542:bool)
          n104 = Select(t=1.0, s=w542, f=-1.0) -> (s? t:f=w539:dbl)
          n105 = Build Array (concatenate)(w545, w539) -> (w538:dbl[])
        }
        n106 = for {
          shift-right: [w530] -> w521
          shift-left: w524 -> [w537]
          tunnel: w523 -> [w536] mode=indexing
          n107 = Greater?(x=w536, y=2.5) -> (0:w534:bool)
          n108 = Select(t=1.0, s=w534, f=-1.0) -> (s? t:f=w531:dbl)
          n109 = Build Array (concatenate)(w537, w531) -> (w530:dbl[])
        }
        n110 = call-poly <vilib>:"CrossCorrelation.vi"("Y"=w521, "X"=w522) -> ("Rxy"=w516:dbl[])  [unwired: 8 in, 1 out]
        n111 = Reciprocal(x=w504) -> (1/x=w517:dbl)
        n112 = Array Max & Min(array=w516) -> (max value=w509:dbl)  [unwired: 3 out]
        n113 = Bundle By Name("Y"=w521, "dt"=w504) -> (w520:waveform(dbl))  [unwired: 1 in]
        n114 = Bundle By Name("Y"=w516, "dt"=w504) -> (w508:waveform(dbl))  [unwired: 1 in]
        n115 = call-poly <vilib>:"FFT Power Spectrum and PSD.vi"("time signal"=w520) -> ("Power Spectrum / PSD"=w507:cluster{"f0":dbl, "df":dbl, "magnitude":dbl[]})  [unwired: 7 in, 3 out]
        n116 = call-poly <vilib>:"FIR Windowed Filter.vi"("sampling freq: fs"=w517, "X"=w516, "filter type"=Filter_Passband_Type."Bandpass", "low cutoff freq: fl"=3000.0, "high cutoff freq: fh"=7000.0, "taps"=256) -> ("Filtered X"=w518:dbl[])  [unwired: 8 in, 1 out]
        n117 = Bundle By Name("Y"=w518, "dt"=w504) -> (w505:waveform(dbl))  [unwired: 1 in]
        n118 = call-poly <vilib>:"FFT Power Spectrum and PSD.vi"("time signal"=w505) -> ("Power Spectrum / PSD"=w506:cluster{"f0":dbl, "df":dbl, "magnitude":dbl[]})  [unwired: 7 in, 3 out]
        n119 = Bundle By Name(cluster=w511, "신호처리[1,-1]"=w508, "신호처리[1,-1][주파수]"=w507, "신호처리[1,-1][필터 후 주파수]"=w506, "신호처리[1,-1][최대값"=w509, "신호처리[1,-1][필터후]"=w505) -> (w510:T4)
      }
      frame "정지" {
        n120 = Release Queue(queue=w549, error in (no error)=w548) -> ()  [unwired: 1 in, 3 out]
        n121 = Release Queue(queue=w547, error in (no error)=w546) -> ()  [unwired: 1 in, 3 out]
        n122 = property on="수신 신호 파형" class="WFGraph (엄격한)"("Val(Sgnl)"=waveform(dbl) {"t0"=timestamp(0 s since 1904-01-01), "dt"=1.0, "Y"=[]} ("Waveform")) -> ()  [unwired: 2 in, 2 out]
        n123 = Unbundle By Name(w556) -> ("AI 참조"=w555:refnum<k21>, "AO 참조"=w554:refnum<k21>, "DO 참조"=w550:refnum<k21>)
        n124 = Equal?(x=w550, y=refnum<k21> refnum) -> (x = y?=w552:bool)
        n125 = case shown="거짓" w552 {
          tunnel: w555 -> [w564 _]
          tunnel: w554 -> [w561 _]
          tunnel: w550 -> [w558 _]
          frame False {
            n126 = call <vilib>:"DAQmx Stop Task.vi"("task/channels in"=w561) -> ("task out"=w562:refnum<k21>, "error out"=w563:errorcluster)  [unwired: 13 in]
            n127 = call <vilib>:"DAQmx Stop Task.vi"("task/channels in"=w564) -> ("task out"=w566:refnum<k21>, "error out"=w565:errorcluster)  [unwired: 13 in]
            n128 = call <vilib>:"DAQmx Stop Task.vi"("task/channels in"=w558) -> ("task out"=w560:refnum<k21>, "error out"=w559:errorcluster)  [unwired: 13 in]
            n129 = call <vilib>:"DAQmx Clear Task.vi"("task in"=w562, "error in"=w563) -> ()  [unwired: 13 in, 1 out]
            n130 = call <vilib>:"DAQmx Clear Task.vi"("task in"=w566, "error in"=w565) -> ()  [unwired: 13 in, 1 out]
            n131 = call <vilib>:"DAQmx Clear Task.vi"("task in"=w560, "error in"=w559) -> ()  [unwired: 13 in, 1 out]
          }
          frame True {
          }
        }
      }
      frame "값 변경" {
        n132 = global read "시작 글로벌.vi" "자동시작 불리언"() -> (w580:bool)
        n133 = case shown="참" w580 {
          tunnel: w579 -> [w590 w593]
          tunnel: w578 -> [w589 w592]
          frame True {
            n134 = Enqueue Element(queue=w590, element=Controller."자동시작" ("원소"), error in (no error)=w589) -> ()  [unwired: 1 in, 3 out]
          }
          frame False {
            n135 = Enqueue Element(queue=w593, element=Controller."수동시작" ("원소"), error in (no error)=w592) -> ()  [unwired: 1 in, 3 out]
          }
        }
        n136 = local read "Mask 길이"() -> (w576:enum16{"8 Order", "12 Order"})
        n137 = local read "Threshold"() -> (w572:u32)
        n138 = local read "Rc"() -> (w569:dbl)
        n139 = local read "수신시간"() -> (w583:dbl)
        n140 = local read "Chip_rate_Threshold"() -> (w574:u32)
        n141 = local read "Mask 데이터 참조 경로"() -> (w582:string)
        n142 = To Double Precision Float(number=w572) -> (double precision float=w571:dbl)
        n143 = To Double Precision Float(number=w574) -> (double precision float=w573:dbl)
        n144 = local read "Version Check"() -> (w567:bool)
        n145 = case shown="\"12 Order\"" w576 {
          tunnel: [256 4096] -> w575
          frame "8 Order", Default {
          }
          frame "12 Order" {
          }
        }
        n146 = call "TXSIG_Generate(SubVi).vi"("Chip_rate_Threshold"=w573, "ThresHold"=w571, "Version 스위치"=w567, "Rc"=w569, "길이"=w575, "이름 또는 상대 경로"=w582) -> ("TXN"=w584:dbl[], "TXP"=w585:dbl[], "TXSIG"=w570:waveform(dbl)[])  [unwired: 3 in]
        n147 = Bundle By Name(cluster=w577, "송신신호 생성"=w570, "TXP 신호"=w585, "TXN 신호"=w584, "Fs"=440000.0, "수신시간"=w583) -> (w581:T4)
      }
      frame "일시정지" {
        n148 = Flush Queue(queue=w605, error in (no error)=w604) -> (queue out=w598:refnum<queue>, error out=w597:errorcluster)  [unwired: 1 out]
        n149 = property on="수신 신호 파형" class="WFGraph (엄격한)"("Val(Sgnl)"=waveform(dbl) {"t0"=timestamp(0 s since 1904-01-01), "dt"=1.0, "Y"=[]} ("Waveform")) -> ()  [unwired: 2 in, 2 out]
        n150 = Unbundle By Name(w599) -> ("AI 참조"=w600:refnum<k21>, "AO 참조"=w601:refnum<k21>, "DO 참조"=w594:refnum<k21>)
        n151 = Enqueue Element(queue=w598, element=Controller."초기화" ("원소"), error in (no error)=w597) -> ()  [unwired: 1 in, 3 out]
        n152 = Equal?(x=w594, y=refnum<k21> refnum) -> (x = y?=w602:bool)
        n153 = case shown="거짓" w602 {
          tunnel: w601 -> [w613 _]
          tunnel: w600 -> [w614 _]
          tunnel: w594 -> [w607 _]
          frame False {
            n154 = call <vilib>:"DAQmx Stop Task.vi"("task/channels in"=w614) -> ("task out"=w612:refnum<k21>, "error out"=w611:errorcluster)  [unwired: 13 in]
            n155 = call <vilib>:"DAQmx Stop Task.vi"("task/channels in"=w613) -> ("task out"=w610:refnum<k21>, "error out"=w609:errorcluster)  [unwired: 13 in]
            n156 = call <vilib>:"DAQmx Stop Task.vi"("task/channels in"=w607) -> ("task out"=w606:refnum<k21>, "error out"=w608:errorcluster)  [unwired: 13 in]
            n157 = call <vilib>:"DAQmx Clear Task.vi"("task in"=w610, "error in"=w609) -> ()  [unwired: 13 in, 1 out]
            n158 = call <vilib>:"DAQmx Clear Task.vi"("task in"=w606, "error in"=w608) -> ()  [unwired: 13 in, 1 out]
            n159 = call <vilib>:"DAQmx Clear Task.vi"("task in"=w612, "error in"=w611) -> ()  [unwired: 13 in, 1 out]
          }
          frame True {
          }
        }
      }
    }
    n160 = Unbundle By Name(w35) -> ("송신신호 생성"=→"송신 신호생성 파형":waveform(dbl)[], "수신 파형"=→"수신 신호 파형":waveform(dbl), "수신 신호처리 파형"=→"신호처리파형":waveform(dbl), "최대값"=→"최대값":dbl, "이전 최대값"=→"이전 최대값":dbl, "최대값 차이"=→"최대값 차이":dbl, "신호처리[1,-1]"=→"신호처리[1.-1]":waveform(dbl), "신호처리[1,-1][최대값"=→"신호처리[1,-1][최대값":dbl, "신호처리[1,-1][주파수]"=→"신호처리[1,-1,][주파수]":cluster{"f0":dbl, "df":dbl, "magnitude":dbl[]}, "신호처리[1,-1][필터 후 주파수]"=→"신호처리[1,-1,][필터후 주파수]":cluster{"f0":dbl, "df":dbl, "magnitude":dbl[]}, "신호처리[1,-1][필터후]"=→"신호처리[1.-1][필터후]":waveform(dbl))
  }
  n161 = while {
    tunnel: w9 -> [w629]
    tunnel: w10 -> [w628]
    shift-right: [w623] -> _
    shift-left: T3 {"연결 ID"=refnum, "TCP 에러"={"status"=FALSE, "code"=0, "source"=""}} -> [w624]
    tunnel: w2 -> [w618]
    tunnel: w1 -> [w617]
    tunnel: [errorcluster {"status"=FALSE, "code"=0, "source"=""} ("에러 상수")] -> w6
    tunnel: [w615] -> w4
    stop <- w625 stop-if-true
    n162 = Dequeue Element(queue=w629, error in (no error)=w628) -> (queue out=w627:refnum<queue>, element=w621:T2, error out=w626:errorcluster)  [unwired: 1 in, 1 out]
    "원소" <- w621
    n163 = Get Queue Status(queue=w618, error in (no error)=w617) -> (queue out=w620:refnum<queue>, error out=w619:errorcluster, # elements in queue=w616:i32)  [unwired: 1 in, 5 out]
    n164 = case shown="\"통신 초기화\", 기본" w621 {
      tunnel: w627 -> [w631 w658 w676]
      tunnel: w626 -> [w630 w657 w675]
      tunnel: [_ _ TRUE] -> w625
      tunnel: w624 -> [w640 w660 w680]
      tunnel: [w639 w659 w677] -> w623
      tunnel: w620 -> [_ w649 _]
      tunnel: w619 -> [_ w648 _]
      tunnel: w616 -> [_ w647 _]
      tunnel: [_ _ w673] -> w615
      frame "통신 초기화", Default {
        w633 = refnum<k5> refnum  # 연결 ID
        n165 = TCP Open Connection(address="주소", remote port or service name="원격 포트 또는 서비스 이름", timeout ms (60000)=1000 ("타임아웃 ms (60000)")) -> (connection ID=w634:refnum<k5>, error out=w636:errorcluster)  [unwired: 2 in]
        n166 = Equal?(x=w634, y=w633) -> (x = y?=w632:bool)
        n167 = Bundle By Name(cluster=w640, "연결 ID"=w634, "TCP 에러"=w636) -> (w639:T3)
        n168 = case shown="참" w632 {
          tunnel: w631 -> [w643 w646]
          tunnel: w630 -> [w642 w645]
          frame False {
            n169 = Enqueue Element(queue=w643, element=DAQ_AO."통신 시작" ("원소"), error in (no error)=w642) -> ()  [unwired: 1 in, 3 out]
          }
          frame True {
            n170 = Enqueue Element(queue=w646, element=DAQ_AO."통신 초기화" ("원소"), error in (no error)=w645) -> ()  [unwired: 1 in, 3 out]
          }
        }
      }
      frame "통신 시작" {
        n171 = Enqueue Element(queue=w658, element=DAQ_AO."통신 시작" ("원소"), error in (no error)=w657) -> ()  [unwired: 1 in, 3 out]
        n172 = Unbundle By Name(w660) -> ("연결 ID"=w653:refnum<k5>, "TCP 에러"=w652:errorcluster)
        n173 = Equal?(x=w647, y=1) -> (x = y?=w655:bool)
        n174 = case shown="참" w655 {
          tunnel: w649 -> [_ w672]
          tunnel: w648 -> [_ w671]
          tunnel: w653 -> [w662 w669]
          tunnel: w652 -> [w661 w668]
          tunnel: [w662 w667] -> w651
          tunnel: [w661 w666] -> w650
          frame False {
          }
          frame True {
            # "4Byte 배열 Packing"
            n175 = Dequeue Element(queue=w672, error in (no error)=w671) -> (element=w664:dbl[])  [unwired: 1 in, 3 out]
            n176 = To Single Precision Float(number=w664) -> (single precision float=w663:sgl[])
            n177 = Type Cast(x=w663) -> (*(type *) &x=w670:string)  [unwired: 1 in]
            n178 = String To Byte Array(string=w670) -> (unsigned byte array=w665:u8[])
            n179 = TCP Write(connection ID=w669, data in=w665, error in (no error)=w668) -> (connection ID out=w667:refnum<k5>, error out=w666:errorcluster)  [unwired: 1 in, 1 out]
            n180 = Array Size(array=w665) -> ()  [unwired: 1 out]
          }
        }
        n181 = Bundle By Name(cluster=w660, "연결 ID"=w651, "TCP 에러"=w650) -> (w659:T3)
      }
      frame "통신 정지" {
        w684 = refnum<k5> refnum  # 연결 ID
        n182 = Release Queue(queue=w676, error in (no error)=w675) -> (error out=w674:errorcluster)  [unwired: 1 in, 2 out]
        n183 = Unbundle By Name(w680) -> ("연결 ID"=w682:refnum<k5>, "TCP 에러"=w681:errorcluster)
        n184 = Merge Errors(w674) -> (w673:errorcluster)
        n185 = Equal?(x=w682, y=w684) -> (x = y?=w683:bool)
        n186 = case shown="참" w683 {
          tunnel: w682 -> [w689 w691]
          tunnel: w681 -> [w688 w690]
          tunnel: [w687 w691] -> w679
          tunnel: [w686 w690] -> w678
          frame False {
            n187 = TCP Close Connection(connection ID=w689, error in (no error)=w688) -> (connection ID out=w687:refnum<k5>, error out=w686:errorcluster)  [unwired: 1 in]
          }
          frame True {
          }
        }
        n188 = Bundle By Name(cluster=w680, "연결 ID"=w679, "TCP 에러"=w678) -> (w677:T3)
      }
    }
  }
  n189 = while {
    tunnel: w17 -> [w700]
    tunnel: w16 -> [w699]
    tunnel: [w697] -> _
    tunnel: [w696] -> _
    tunnel: w9 -> [w695]
    tunnel: w10 -> [w694]
    tunnel: [w693] -> _
    tunnel: [w692] -> _
    stop <- w698 stop-if-true
    n190 = event shown="[1] \"수동시작 버튼\": 값 변경" {
      selector: _ -> [_ _ _ _]
      dyn-events: _ -> [_ _ _ _]
      timeout: _ -> [_ _ _ _]
      tunnel: w700 -> [w710 w721 w726 w733]
      tunnel: w699 -> [w711 w722 w727 w734]
      tunnel: [TRUE _ _ _] -> w698
      tunnel: [w713 w716 w723 w728] -> w697
      tunnel: [w712 w717 w724 w729] -> w696
      tunnel: w695 -> [w704 _ _ _]
      tunnel: w694 -> [w703 _ _ _]
      tunnel: [w702 _ _ _] -> w693
      tunnel: [w701 _ _ _] -> w692
      event "정지 버튼": Value Change {
        n191 = event-data() -> ()  [unwired: 1 in, 1 out]
        n192 = Flush Queue(queue=w711, error in (no error)=w710) -> (queue out=w709:refnum<queue>, error out=w708:errorcluster)  [unwired: 1 out]
        n193 = Flush Queue(queue=w704, error in (no error)=w703) -> (queue out=w707:refnum<queue>, error out=w706:errorcluster)  [unwired: 1 out]
        n194 = Enqueue Element(queue=w709, element=Controller."정지" ("원소"), error in (no error)=w708) -> (queue out=w712:refnum<queue>, error out=w713:errorcluster)  [unwired: 1 in, 1 out]
        n195 = Enqueue Element(queue=w707, element=DAQ_AO."통신 정지" ("원소"), error in (no error)=w706) -> (queue out=w702:refnum<queue>, error out=w701:errorcluster)  [unwired: 1 in, 1 out]
      }
      event "수동시작 버튼": Value Change {
        n196 = event-data() -> ()  [unwired: 1 in, 1 out]
        n197 = Enqueue Element(queue=w722, element=Controller."값 변경" ("원소"), error in (no error)=w721) -> (queue out=w717:refnum<queue>, error out=w716:errorcluster)  [unwired: 1 in, 1 out]
        n198 = global write "시작 글로벌.vi" "자동시작 불리언"(FALSE) -> ()
        n199 = global write "시작 글로벌.vi" "수동시작 불리언"(TRUE) -> ()
      }
      event "일시 정지 버튼": Value Change {
        n200 = event-data() -> ()  [unwired: 1 in, 1 out]
        n201 = Enqueue Element(queue=w727, element=Controller."일시정지" ("원소"), error in (no error)=w726) -> (queue out=w724:refnum<queue>, error out=w723:errorcluster)  [unwired: 1 in, 1 out]
      }
      event "자동시작 버튼": Value Change {
        n202 = event-data() -> ()  [unwired: 1 in, 1 out]
        n203 = Enqueue Element(queue=w734, element=Controller."값 변경" ("원소"), error in (no error)=w733) -> (queue out=w729:refnum<queue>, error out=w728:errorcluster)  [unwired: 1 in, 1 out]
        n204 = global write "시작 글로벌.vi" "자동시작 불리언"(TRUE) -> ()
        n205 = global write "시작 글로벌.vi" "수동시작 불리언"(FALSE) -> ()
      }
    }
  }
  n206 = Merge Errors(w6, w4) -> (w5:errorcluster)
  n207 = Merge Errors(w3, w5) -> (w7:errorcluster)
  n208 = call <vilib>:"General Error Handler.vi"("error in (no error)"=w7) -> ()  [unwired: 10 in, 5 out]
